vi "Focus Set Home Bit.vi"(8 "error in (no error)":errorcluster, 9 "Homed?":bool, 10 "Motor (0:n-1)":i32, 11 "Focus Class in":refnum<class "Focus Class.lvclass">) -> (0 "error out":errorcluster, 3 "Focus Class out":refnum<class "Focus Class.lvclass">)   [LabVIEW 2024, in "Focus Class.lvclass"]
uses:
  Focus Class.lvclass
  Focus Class.lvclass/Focus Class.ctl
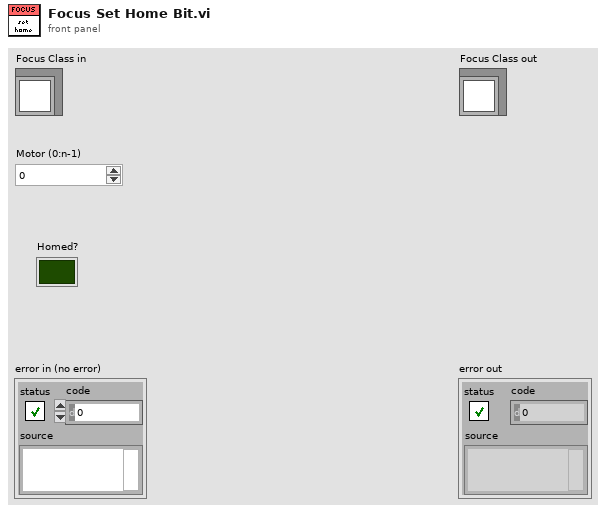
[diagram p1: front panel]
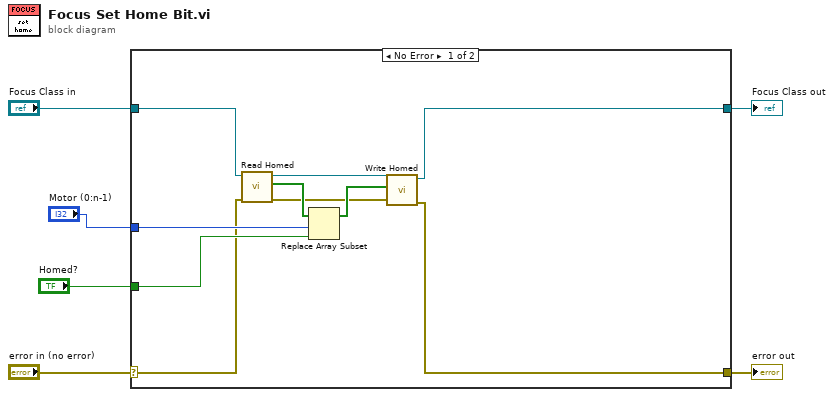
[diagram p0: block diagram]
diagram:
  n1 = case shown="No Error" "error in (no error)" {
    selector: "error in (no error)" -> [w11 w18]
    tunnel: [w9 w18] -> w5
    tunnel: [w8 w17] -> w3
    tunnel: "Focus Class in" -> [w7 w17]
    tunnel: "Motor (0:n-1)" -> [w14 _]
    tunnel: "Homed?" -> [w13 _]
    frame No Error {
      n2 = call "Read Homed.vi"("error in (no error)"=w11, "Focus Class in"=w7) -> ("error out"=w10:errorcluster, "Homed"=w15:bool[], "Focus Class out"=w16:refnum<class "Focus Class.lvclass">)  [unwired: 7 in]
      n3 = Replace Array Subset(array=w15, new element=w13, index=w14) -> (w12:bool[])
      n4 = call "Write Homed.vi"("error in (no error)"=w10, "Homed"=w12, "Focus Class in"=w16) -> ("error out"=w9:errorcluster, "Focus Class out"=w8:refnum<class "Focus Class.lvclass">)  [unwired: 7 in]
    }
    frame Error {
    }
  }
  "error out" <- w5
  "Focus Class out" <- w3
